vi "Write Control Limits - All.vi"(8 "error in (no error)":errorcluster, 10 "control limits":T1={"Limit Low"=variant(dbl 0.0), "Limit High"=variant(dbl 0.0), "Min Step"=variant(dbl 0.0)}, 11 "NT Scalar (Numeric) in":refnum<class "NT Scalar (Numeric).lvclass">) -> (0 "error out":errorcluster, 3 "NT Scalar (Numeric) out":refnum<class "NT Scalar (Numeric).lvclass">)   [LabVIEW 2020, in "PV Access.lvlib" / "PV Data.lvlib" / "NT Scalar (Numeric).lvclass"]
uses:
  NT Scalar (Numeric).lvclass
  NT Scalar (Numeric).lvclass/NT Scalar (Numeric).ctl
  Control Metadata.ctl
  PV Data.lvlib
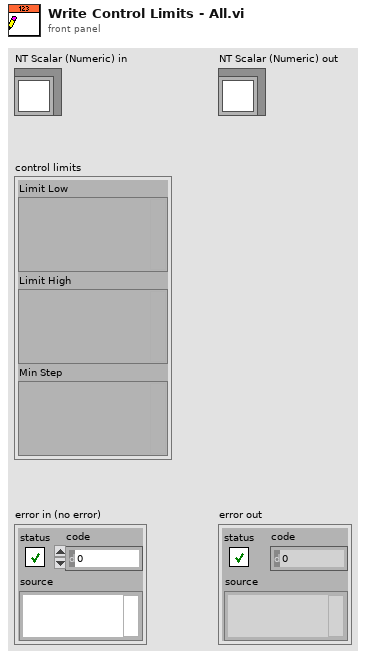
[diagram p1: front panel]
types:
  T1 = typedef "PV Access.lvlib/PV Data.lvlib/Control Metadata.ctl" = cluster{"Limit Low":variant, "Limit High":variant, "Min Step":variant}
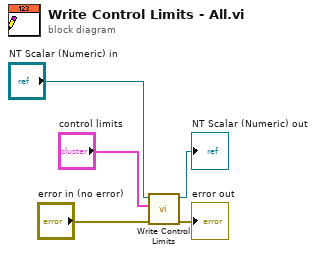
[diagram p0: block diagram]
diagram:
  n1 = call-dynamic "Write Control Limits.vi"("error in"="error in (no error)", "control limits"="control limits", "Has Control Limits in"="NT Scalar (Numeric) in") -> ("error out"=→"error out":errorcluster, "Has Control Limits out"=→"NT Scalar (Numeric) out":refnum<class "NT Scalar (Numeric).lvclass">)  [unwired: 7 in]
